vi "encoder.vi"(1 "Command input":cluster{"Command":string, "Payload":sgl}={"Command"="", "Payload"=1.0}) -> (0 "Command string":string)   [LabVIEW 2020]
panel:
  out "data string":string
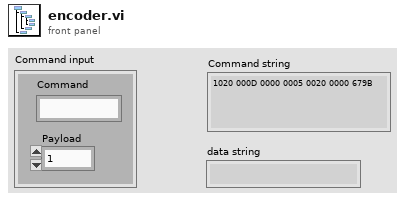
[diagram p1: front panel]
types:
  T1 = enum16{"big-endian, network order", "native, host order", "little-endian"}
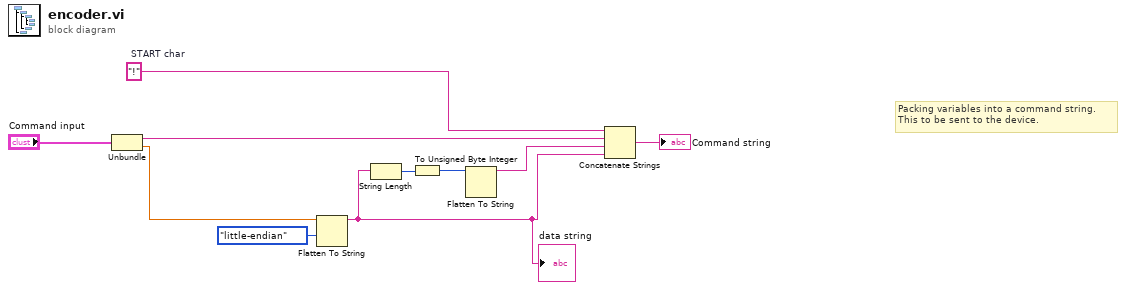
[diagram p0: block diagram]
diagram:
  w8 = "!"  # START char
  # "Packing variables into a command string.\nThis to be sent to the device."
  n1 = Unbundle("Command input") -> ("Command"=w7:string, "Payload"=w1:sgl)
  n2 = Flatten To String(anything=w1, byte order (0:big-endian, network order)=T1."little-endian") -> (data string=w2:string)  [unwired: 2 in, 2 out]
  "data string" <- w2
  n3 = String Length(string=w2) -> (length=w6:i32)
  n4 = To Unsigned Byte Integer(number=w6) -> (unsigned 8bit integer=w5:u8)
  n5 = Flatten To String(anything=w5) -> (data string=w4:string)  [unwired: 3 in, 2 out]
  n6 = Concatenate Strings(w8, w7, w4, w2) -> (→"Command string":string)
